vi "Excel Set Cell Color and Border.vi"(0 "report in":refnum<class "NI_report.lvclass">, 1 "inside border":T1={"on/off"=FALSE, "weight"=2, "color"=0} {"weight" items=["xlHairline"=1, "xlMedium"=-4138, "xlThick"=4, "xlThin"=2]}, 2 "outside border":T1={"on/off"=FALSE, "weight"=2, "color"=0} {"weight" items=["xlHairline"=1, "xlMedium"=-4138, "xlThick"=4, "xlThin"=2]}, 5 "background color (w)":u32(colorbox)=16777215, 7 "start (-1, -1)":cluster{"row":i32, "column":i32}={"row"=-1, "column"=-1}, 9 "end (-1, -1)":cluster{"row":i32, "column":i32}={"row"=-1, "column"=-1}, 11 "error in (no error)":errorcluster, 12 "name (\"\")":string) -> (4 "report out":refnum<class "NI_report.lvclass">, 15 "error out":errorcluster)   [LabVIEW 2010, in "NI_Excel.lvclass"]
doc: "Sets the borders and background color of the cells specified by the <B>start</B> and <B>end</B> clusters or by a named range."
uses:
  <vilib>/Utility/NIReport.llb/Excel/NI_Excel.lvclass
  <vilib>/Utility/NIReport.llb/NI_report.lvclass
  <vilib>/Utility/NIReport.llb/Excel/NI_Excel.lvclass/NI_Excel.ctl
  NI_ReportGenerationToolkit.lvlib
  <vilib>/Utility/NIReport.llb/NI_ReportGenerationCore.lvlib
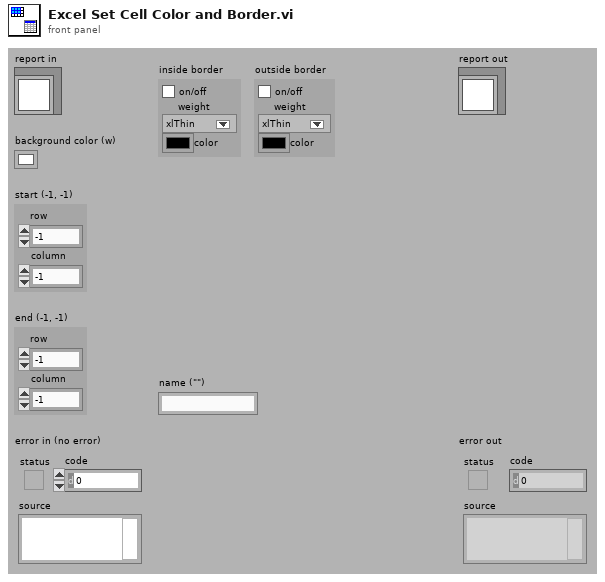
[diagram p1: front panel]
types:
  T1 = cluster{"on/off":bool, "weight":i32, "color":u32}
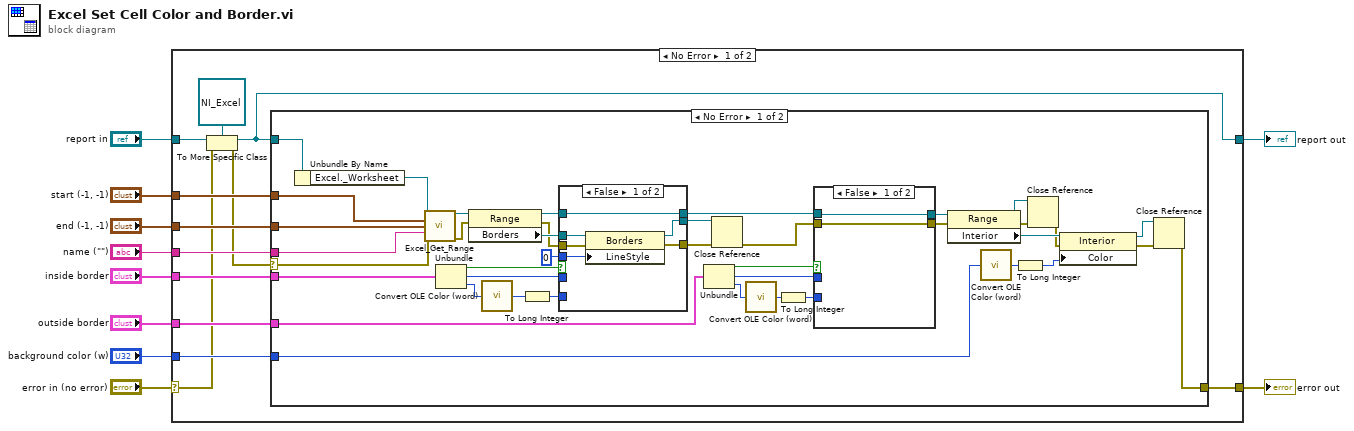
[diagram p0: block diagram]
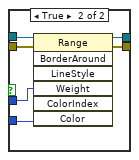
[diagram p2: hidden frame]
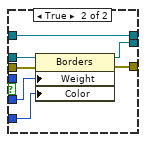
[diagram p3: hidden frame]
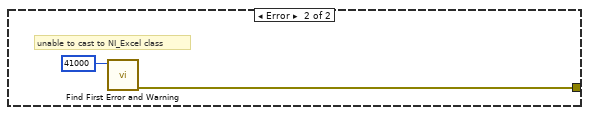
[diagram p4: hidden frame]
diagram:
  n1 = case shown="No Error" "error in (no error)" {
    selector: "error in (no error)" -> [w11 w87]
    tunnel: [w16 w87] -> w9
    tunnel: [w13 w86] -> w7
    tunnel: "report in" -> [w14 w86]
    tunnel: "start (-1, -1)" -> [w22 _]
    tunnel: "end (-1, -1)" -> [w21 _]
    tunnel: "name (\"\")" -> [w20 _]
    tunnel: "inside border" -> [w19 _]
    tunnel: "outside border" -> [w18 _]
    tunnel: "background color (w)" -> [w17 _]
    frame No Error {
      n2 = To More Specific Class(target class=refnum<class "NI_Excel.lvclass"> refnum ("report in"), reference=w14, error in=w11) -> (specific class reference=w13:refnum<class "NI_Excel.lvclass">, error out=w12:errorcluster)
      n3 = case shown="No Error" w12 {
        selector: w12 -> [w23 _]
        tunnel: w13 -> [w32 _]
        tunnel: w22 -> [w31 _]
        tunnel: w21 -> [w30 _]
        tunnel: w20 -> [w29 _]
        tunnel: w19 -> [w28 _]
        tunnel: w18 -> [w27 _]
        tunnel: w17 -> [w26 _]
        tunnel: [w25 w84] -> w16
        frame No Error {
          n4 = Unbundle By Name(w32) -> ("Excel._Worksheet"=w24:refnum<k7>)
          n5 = call <vilib>:"Excel_Get_Range.vi"("Excel._Worksheet"=w24, "start"=w31, "end"=w30, "name"=w29, "error in (no error)"=w23) -> ("Range"=w57:refnum<k7>, "error out"=w58:errorcluster)  [unwired: 5 in, 4 out]
          n6 = Unbundle(w28) -> ("on/off"=w51:bool, "weight"=w49:i32, "color"=w48:u32)
          n7 = property class="Range"(reference=w57, error in=w58) -> (reference out=w52:refnum<k7>, error out=w42:errorcluster, "Borders"=w50:refnum<k7>)
          n8 = call <vilib>:"Convert OLE Color (word).vi"("color in"=w48) -> ("color out"=w34:u32)
          n9 = To Long Integer(number=w34) -> (32bit integer=w59:i32)
          n10 = case shown="False" w51 {
            tunnel: w59 -> [_ w83]
            tunnel: [w72 w82] -> w40
            tunnel: [w74 w81] -> w41
            tunnel: w42 -> [w75 w80]
            tunnel: w49 -> [_ w79]
            tunnel: w50 -> [w73 w78]
            tunnel: w52 -> [w76 w77]
            tunnel: [w76 w77] -> w53
            tunnel: 0 -> [w71 _]
            frame False {
              n11 = property class="Borders"(reference=w73, error in=w75, "LineStyle"=w71) -> (reference out=w72:refnum<k7>, error out=w74:errorcluster)
            }
            frame True {
              n12 = property class="Borders"(reference=w78, error in=w80, "Weight"=w79, "Color"=w83) -> (reference out=w82:refnum<k7>, error out=w81:errorcluster)
            }
          }
          n13 = Unbundle(w27) -> ("on/off"=w56:bool, "weight"=w55:i32, "color"=w54:u32)
          n14 = Close Reference(reference=w40, error in (no error)=w41) -> (error out=w44:errorcluster)
          n15 = call <vilib>:"Convert OLE Color (word).vi"("color in"=w54) -> ("color out"=w47:u32)
          n16 = To Long Integer(number=w47) -> (32bit integer=w60:i32)
          n17 = case shown="False" w56 {
            tunnel: w44 -> [w63 w70]
            tunnel: [w63 w69] -> w45
            tunnel: [w64 w68] -> w46
            tunnel: w60 -> [_ w67]
            tunnel: w53 -> [w64 w66]
            tunnel: w55 -> [_ w65]
            frame False {
            }
            frame True {
              n18 = invoke class="Range" method="BorderAround"(reference=w66, error in=w70, "Weight"=w65, "Color"=w67) -> (reference out=w68:refnum<k7>, error out=w69:errorcluster)  [unwired: 3 in, 5 out]
            }
          }
          n19 = property class="Range"(reference=w46, error in=w45) -> (reference out=w36:refnum<k7>, error out=w38:errorcluster, "Interior"=w43:refnum<k7>)
          n20 = call <vilib>:"Convert OLE Color (word).vi"("color in"=w26) -> ("color out"=w33:u32)
          n21 = To Long Integer(number=w33) -> (32bit integer=w61:i32)
          n22 = Close Reference(reference=w36, error in (no error)=w38) -> (error out=w37:errorcluster)
          n23 = property class="Interior"(reference=w43, error in=w37, "Color"=w61) -> (reference out=w35:refnum<k7>, error out=w39:errorcluster)
          n24 = Close Reference(reference=w35, error in (no error)=w39) -> (error out=w25:errorcluster)
        }
        frame Error {
          # "unable to cast to NI_Excel class"
          n25 = call <vilib>:"Find First Error and Warning.vi"("error code"=41000) -> ("error out"=w84:errorcluster)  [unwired: 2 in, 4 out]
        }
      }
    }
    frame Error {
    }
  }
  "error out" <- w9
  "report out" <- w7
